vi "ServidorTCP_17_05.vi"() -> ()   [LabVIEW 2020]
uses:
  <vilib>/Platform/TimedLoop/XDataNode/timing_clust.ctl
  <vilib>/Platform/TimedLoop/XDataNode/nitl_modes.ctl
  <vilib>/Platform/TimedLoop/XDataNode/wakeup.ctl
  <vilib>/Instr/_visa.llb/VISA Configure Serial Port (Instr).vi
  <vilib>/Platform/TimedLoop/XDataNode/XDataNode.xnode
  <vilib>/Platform/TimedLoop/XDataNode/XDNodeRunTimeDep.lvlib
panel:
  in  "mode (standard)":T1(ring)
  in  "bytes to read":i32
  out "PWM":i32(graph)
  out "Iluminación":u32(graph)
  out "longitud buffer":i32
  out "x = y?":bool
  out "bytes enviados TCP":i32
  out "DentroWhile":string
  out "buffer":string
  in  "Direccion IP del cliente":string
  in  "Puerto":u16
  in  "Puerto COM":refnum<visa-resource-name>
  # "SERVIDOR"
  # "COMUNICACION Serie"
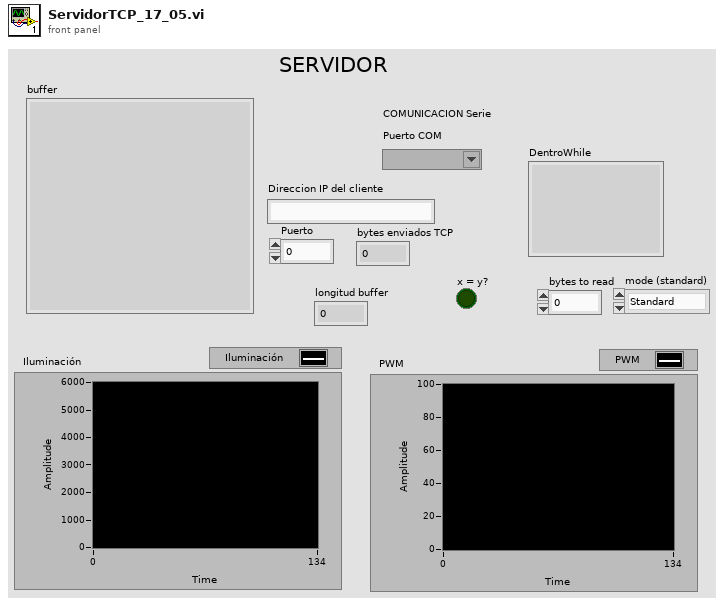
[diagram p1: front panel]
types:
  T1 = enum16{"Standard", "Buffered", "CRLF", "Immediate"}
  T2 = typedef "XDNodeRunTimeDep.lvlib/timing_clust.ctl" = cluster{"Expected End [f-1]":u64, "Actual End [f-1]":u64, "Finished Late? [f-1]":bool, "Expected End [i-1]":u64, "Actual End [i-1]":u64, "Finished Late? [i-1]":bool, "Expected Start [i]":u64, "Actual Start [i]":u64, "Expected Start [f]":u64, "Actual Start [f]":u64, "Source Name":string, "Structure Name":string, "Period":i64, "Deadline":i64, "Offset":i64, "Start":i64, "Priority":i32, "Timeout":i32, "Mode":T3, "Wakeup Reason":T4, "Error":errorcluster, "Source Type":string, "Secondary Source Type":string, "Global End Time":u64, "Global Start Time":u64, "Frame Duration":u64, "Iteration Duration":u64, "Assigned CPU":i32, "I/O Scan Engine Mode":u32}
  T3 = typedef "XDNodeRunTimeDep.lvlib/nitl_modes.ctl" = enum32{"No Change", "Process missed periods, maintain original phase", "Discard missed periods, maintain original phase", "Process missed periods, ignore original phase", "Discard missed periods, ignore original phase"}
  T4 = typedef "XDNodeRunTimeDep.lvlib/wakeup.ctl" = enum32{"Normal", "Aborted", "Asynchronous wakeup", "Timing source error", "Timed loop error", "Timeout"}
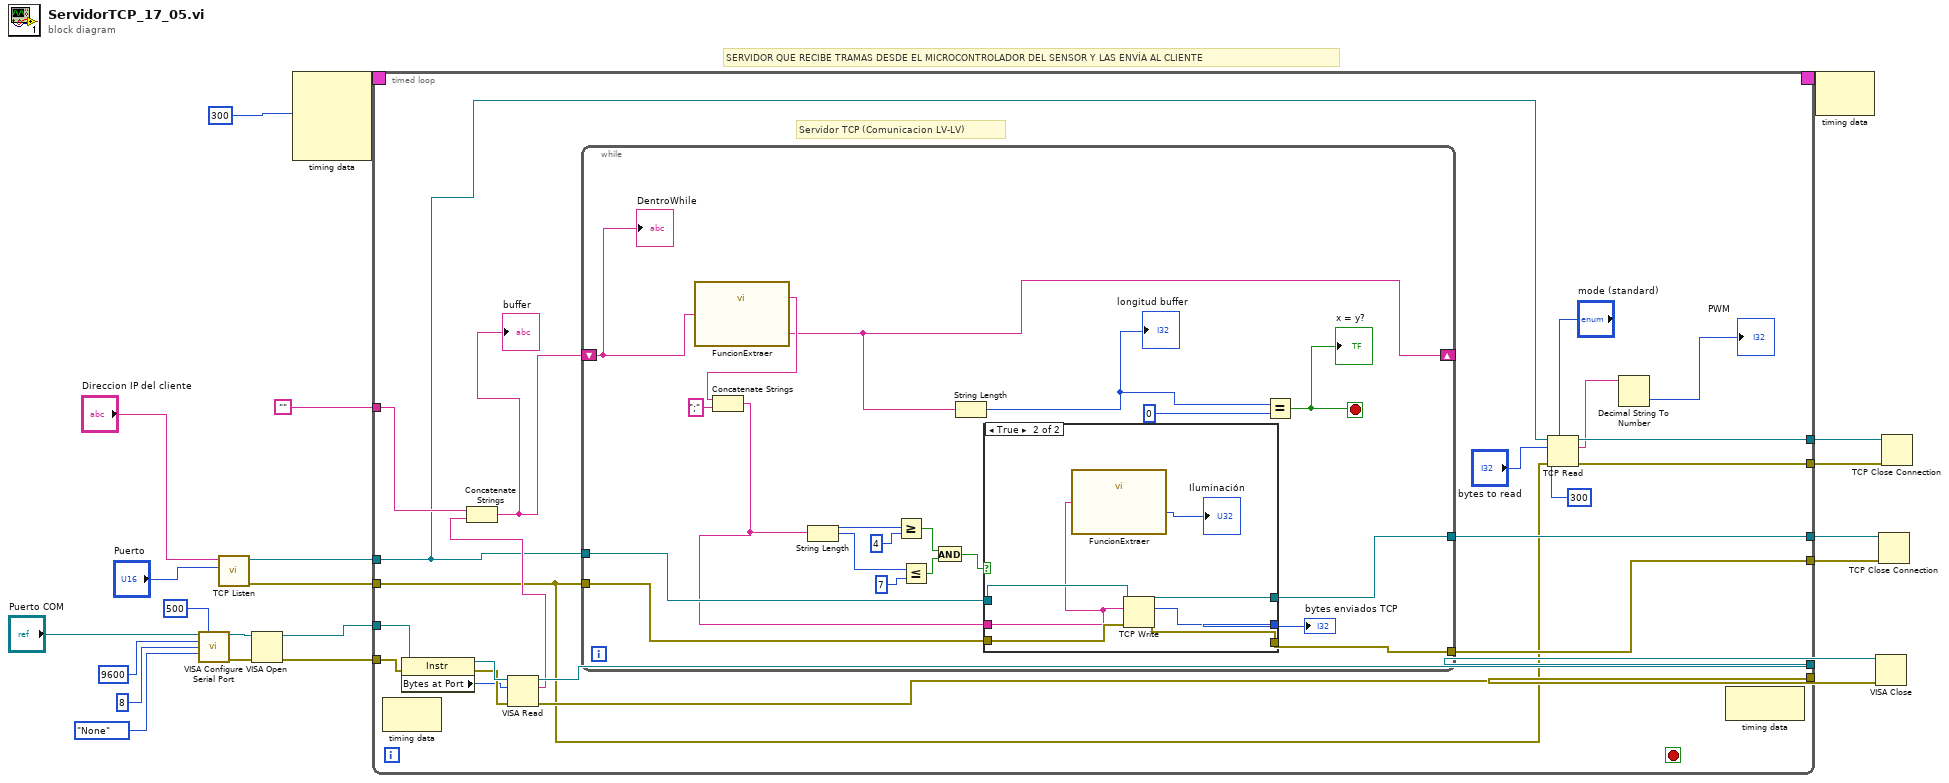
[diagram p0: block diagram]
diagram:
  # "SERVIDOR QUE RECIBE TRAMAS DESDE EL MICROCONTROLADOR DEL SENSOR Y LAS ENVÍA AL CLIENTE"
  n1 = call-poly "VISA Configure Serial Port"("VISA resource name"="Puerto COM", "timeout (10sec)"=u32 500, "baud rate (9600)"=u32 9600, "data bits (8)"=u16 8, "parity (0:none)"=enum16{"None", "Odd", "Even", "Mark", "Space"}."None") -> ("VISA resource name out"=w16:refnum<visa-resource-name>, "error out"=w15:errorcluster)  [unwired: 9 in]
  n2 = call <vilib>:"TCP Listen.vi"("port"="Puerto", "service name"="Direccion IP del cliente") -> ("error out"=w7:errorcluster, "connection ID"=w1:refnum<k5>)  [unwired: 5 in, 3 out]
  n3 = VISA Open(error in (no error)=w15, VISA resource name=w16) -> (VISA resource name=w9:refnum<visa-resource-name>, error out=w10:errorcluster)  [unwired: 3 in]
  n4 = node-c288(i64 300 ("Period")) -> (w23:T2)  [unwired: 3 in]
  n5 = timed-loop {
    timing: w23 -> [_]
    timing-out: [_] -> w22
    tunnel: [w40] -> w11
    tunnel: w10 -> [w39]
    tunnel: w9 -> [w38]
    tunnel: [w37] -> w8
    tunnel: w7 -> [w27]
    tunnel: w1 -> [w26]
    tunnel: [w36] -> w6
    tunnel: [w35] -> w5
    tunnel: "" -> [w33]
    tunnel: [w32] -> w3
    tunnel: [w31] -> w2
    stop <- _ stop-if-true
    # "Servidor TCP (Comunicacion LV-LV)"
    n6 = node-c288() -> ()  [unwired: 1 in, 1 out]
    n7 = property class="Instr"(reference=w38, error in=w39) -> (reference out=w44:refnum<visa-resource-name>, error out=w43:errorcluster, "Bytes at Port"=w42:u32)
    n8 = VISA Read(VISA resource name=w44, byte count=w42, error in (no error)=w43) -> (VISA resource name out=w37:refnum<visa-resource-name>, read buffer=w34:string, error out=w40:errorcluster)  [unwired: 1 out]
    n9 = Concatenate Strings(w33, w34) -> (w41:string)
    "buffer" <- w41
    n10 = while {
      tunnel: w27 -> [w63]
      tunnel: w26 -> [w62]
      tunnel: [w45] -> w36
      tunnel: [w61] -> w35
      shift-right: [w53] -> _
      shift-left: w41 -> [w56]
      stop <- w57 stop-if-true
      n11 = call "FuncionExtraer.vi"("Buffer entrada"=w56) -> ("Mensaje sin \";\""=w54:string, "Mensaje restante"=w53:string)  [unwired: 5 in, 4 out]
      n12 = Concatenate Strings(w54, ";" ("string")) -> (w52:string)
      n13 = String Length(string=w52) -> (length=w50:i32)
      n14 = Greater Or Equal?(x=w50, y=4) -> (x >= y?=w48:bool)
      n15 = Less Or Equal?(x=w50, y=7) -> (x <= y?=w47:bool)
      n16 = And(x=w48, y=w47) -> (x .and. y?=w46:bool)
      n17 = String Length(string=w53) -> (length=w59:i32)
      "longitud buffer" <- w59
      n18 = case shown="True" w46 {
        tunnel: w63 -> [_ w70]
        tunnel: w62 -> [_ w69]
        tunnel: [_ w68] -> w45
        tunnel: [_ w67] -> w61
        tunnel: [_ w66] -> w60
        tunnel: w52 -> [_ w65]
        frame False {
        }
        frame True {
          n19 = call "FuncionExtraer.vi"("Buffer entrada"=w65) -> ("lux (decimal)"=→"Iluminación":u32)  [unwired: 5 in, 5 out]
          n20 = TCP Write(connection ID=w69, data in=w65, error in (no error)=w70) -> (connection ID out=w68:refnum<k5>, bytes written=w66:i32, error out=w67:errorcluster)  [unwired: 1 in]
        }
      }
      "bytes enviados TCP" <- w60
      n21 = Equal?(x=w59, y=0) -> (x = y?=w57:bool)
      "x = y?" <- w57
      "DentroWhile" <- w56
    }
    n22 = TCP Read(connection ID=w26, bytes to read="bytes to read", error in (no error)=w27, 7:"mode (standard)", 9:300 ("timeout ms (25000)")) -> (connection ID out=w32:refnum<k5>, data out=w30:string, error out=w31:errorcluster)
    n23 = Decimal String To Number(string=w30) -> (number=→"PWM":i32)  [unwired: 2 in, 1 out]
    n24 = node-c288() -> ()  [unwired: 1 in, 1 out]
  }
  n25 = node-c288(w22) -> ()  [unwired: 1 out]
  n26 = VISA Close(VISA resource name=w8, error in (no error)=w11) -> ()  [unwired: 1 out]
  n27 = TCP Close Connection(connection ID=w6, error in (no error)=w5) -> ()  [unwired: 1 in, 2 out]
  n28 = TCP Close Connection(connection ID=w3, error in (no error)=w2) -> ()  [unwired: 1 in, 2 out]
